vi "Get Sequence Call Info.vi"(8 "error in (no error)":errorcluster, 10 "Sequence Name":string, 11 "Session Ref in":T2) -> (0 "error out":errorcluster, 1 "Sequence Call Ref":T1, 2 "Sequence Name out":string, 3 "Session Ref out":T2)   [LabVIEW 2020, in "NI_VS Sequence Execution Interface.lvlib"]
doc: "Returns a sequence call refnum for a real-time sequence in an NI VeriStand stimulus profile session."
uses:
  <vilib>/NI VeriStand/Execution/SequenceExecutionInterface/NI_VS Sequence Execution Interface.lvlib
  <vilib>/NI VeriStand/Execution/SequenceExecutionInterface/Stimulus Profile Session Ref.ctl
  NationalInstruments.VeriStand.ClientAPI
  <vilib>/NI VeriStand/Execution/SequenceExecutionInterface/Sequence Call Ref.ctl
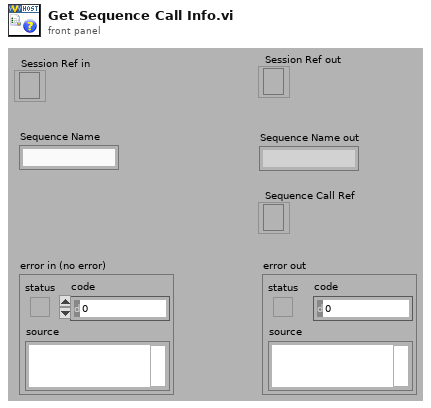
[diagram p1: front panel]
types:
  T1 = typedef "NI_VS Sequence Execution Interface.lvlib/Sequence Call Ref.ctl" = refnum<k24>
  T2 = typedef "NI_VS Sequence Execution Interface.lvlib/Stimulus Profile Session Ref.ctl" = refnum<k24>
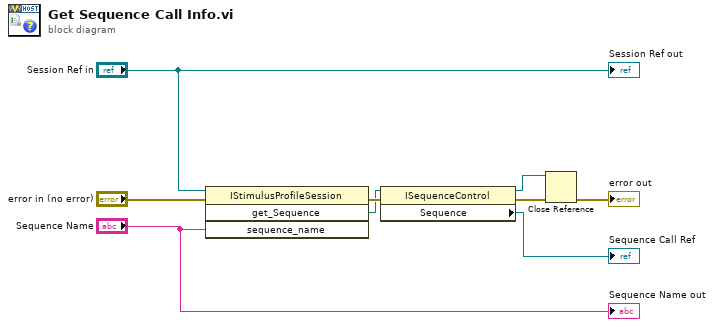
[diagram p0: block diagram]
diagram:
  n1 = invoke class="IStimulusProfileSession" method="get_Sequence"(reference="Session Ref in", error in="error in (no error)", "sequence_name"="Sequence Name") -> (error out=w6:errorcluster, "get_Sequence"=w5:refnum<k24>)  [unwired: 1 in, 2 out]
  n2 = property class="ISequenceControl"(reference=w5, error in=w6) -> (reference out=w4:refnum<k24>, error out=w3:errorcluster, "Sequence"=→"Sequence Call Ref":refnum<k24>)
  n3 = Close Reference(reference=w4, error in (no error)=w3) -> (error out=→"error out":errorcluster)
  "Session Ref out" <- "Session Ref in"
  "Sequence Name out" <- "Sequence Name"
